vi "Demo - Advanced Use.vi"() -> ()   [LabVIEW 2013, in "GOLPI library.lvlib"]
doc: "Very simple demonstration of use of the GOLPI library.\n\n---\nGOLPI works only with lv_proc.dll library, which is part of vipm package or should be delivered together with packed library. Placement of this dll is selected in terminal of Start GNU Octave.vi."
uses:
  GOLPI library.lvlib
  Private/Set Variable - polymorph parts/Set Double Complex.vi
  Private/Get Variable - polymorph parts/Get Double.vi
panel:
  in  "octave exe file or directory":path=path "C:/Octave/Octave-4.0.0/bin"
  out "exit code of GNU\nOctave process:":i32
  out "One can see all writings to stdin or readings\nfrom stdout if debug mode was enabled:":string
  in  "timeout of this reading is":u32=14000 format="%_2p"
  out "LabVIEW now waited":u32
  in  "And wait till one of following\nkeywords appears:":string[](array[string])=["error", "demokeyword"]
  in  "Try again this time consuming\ncalculation without output:":string="for i=[1:10]\n   pause(1)\nendfor\ndisp('demokeyword')"
  out "parse error":errorcluster
  out "syntax error":errorcluster
  in  "Lets try this parse error:":string="disp()"
  in  "Lets try this syntax error:":string="sin('aa'))"
  in  "and the value of variable":string="R"
  out "LabVIEW waited":u32
  in  "timeout of all reading is":u32=14000 format="%_2p"
  in  "And read output till is settled for":u32=1200 format="%_2p"
  in  "Try this time consuming calculation:":string="for i=[1:10]\n   pause(1)\n   disp(i)\nendfor"
  out "is":dbl format="%.2f"
  in  "then calculate this equation:":string="R=abs(sqrt(Z))"
  in  "Set this value":cdb=32.56-126.3i
  in  "to a variable named":string="Z"
  out "error out":errorcluster
  in  "working directory":path=path "C:/"
  # "Writing and reading value with GOLPI Set/Get vis"
  # "How GOLPI reacts to GNU Octave syntax error"
  # ","
  # ","
  # "."
  # "Wait for GNU Octave with 'Read Output till settle.vi'"
  # "ms,"
  # "ms."
  # "ms."
  # "How GOLPI reacts to GNU Octave parse error"
  # "Wait with 'Read Output till Keyword.vi'"
  # "ms."
  # "ms."
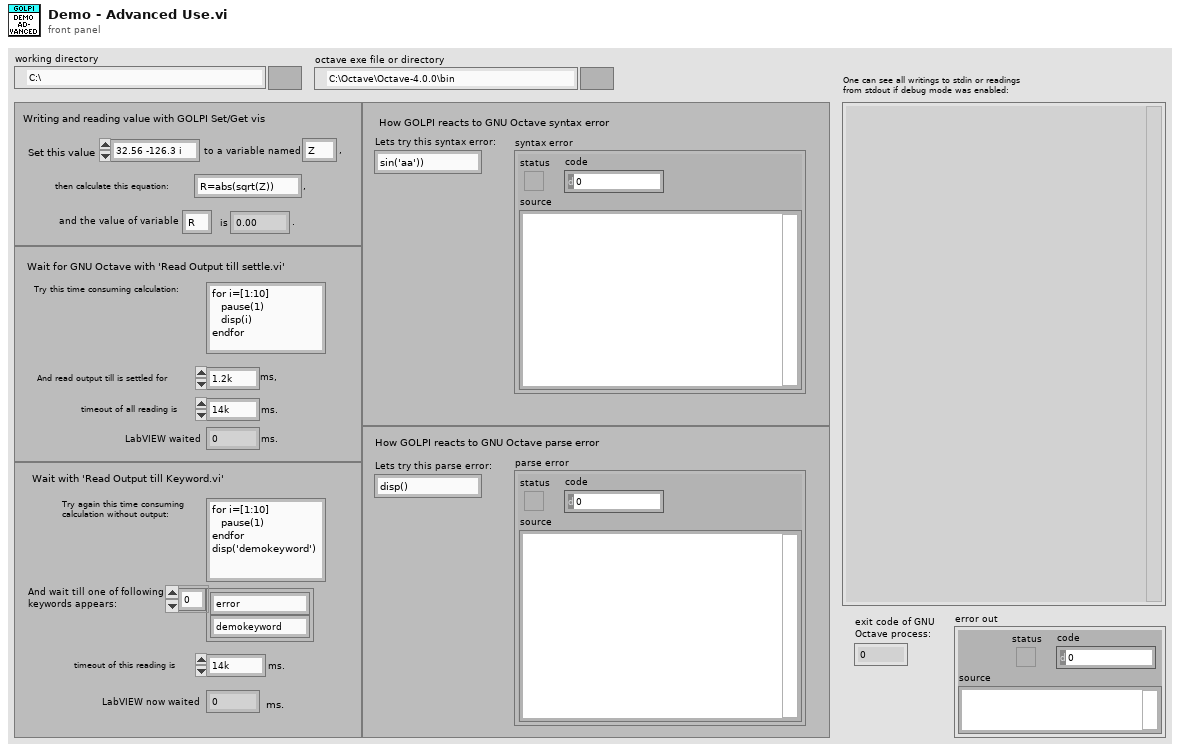
[diagram p1: front panel]
types:
  T1 = typedef "GOLPI library.lvlib/GOLPI reference Type Def.ctl" = cluster{"pipe handle":T2, "fast read timeout [ms]":u32, "fast read settle time [ms]":u32, "fast read to multiple [ms]":u32, "max elements per input line":u32, "slow read timeout [ms]":u32, "stdin double format specifier":string, "max elements per stdout output column":u32}
  T2 = typedef "LV Process library.lvlib/Pipe Handle.ctl" = cluster{"lv_proc.dll file path":path, "process instance handle":u32[], "debug mode":bool, "debug data":cluster{"time":timestamp, "stdin":bool, "data":string}[]}
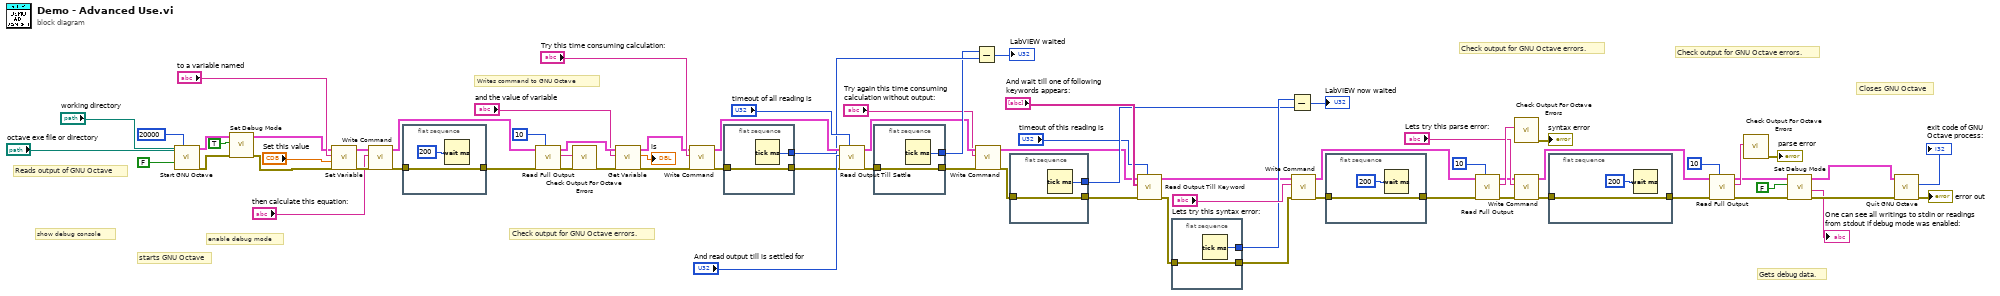
[diagram p0: block diagram]
diagram:
  # "Gets debug data."
  # "Check output for GNU Octave errors."
  # "Check output for GNU Octave errors."
  # "show debug console"
  # "enable debug mode"
  # "Check output for GNU Octave errors."
  # "Closes GNU Octave"
  # "Reads output of GNU Octave"
  # "Writes command to GNU Octave"
  # "starts GNU Octave"
  n1 = call "Start GNU Octave.vi"("working directory"="working directory", "full start timeout [ms] (20000)"=u32 20000 ("Full start timeout [ms] (5000)"), "octave exe file or directory"="octave exe file or directory", "hide debug console (T)"=FALSE) -> ("GOLPI ref. out"=w35:T1, "error out"=w3:errorcluster)  [unwired: 8 in, 2 out]
  n2 = call "Set Debug Mode.vi"("error in"=w3, "debug mode (F)"=TRUE, "GOLPI ref. in"=w35) -> ("error out"=w2:errorcluster, "GOLPI ref. out"=w34:T1)  [unwired: 5 in, 2 out]
  n3 = call-poly "Set Variable.vi"("error in"=w2, "value"="Set this value", "variable name"="to a variable named", "GOLPI ref. in"=w34) -> ("error out"=w70:errorcluster, "GOLPI ref. out"=w71:T1)  [unwired: 6 in]
  n4 = call "Write Command.vi"("error in"=w70, "command"="then calculate this equation:", "GOLPI ref. in"=w71) -> ("error out"=w28:errorcluster, "GOLPI ref. out"=w27:T1)  [unwired: 7 in]
  n5 = flat-sequence {
    tunnel: [w75] -> w29
    tunnel: w28 -> [w75]
    frame #0 {
      n6 = Wait (ms)(milliseconds to wait=u32 200) -> ()  [unwired: 1 out]
    }
  }
  n7 = call "Read Full Output.vi"("timeout [ms]"=u32 10, "error in"=w29, "GOLPI ref. in"=w27) -> ("error out"=w64:errorcluster, "read buffer"=w62:string, "GOLPI ref. out"=w63:T1)  [unwired: 5 in, 1 out]
  n8 = call "Check Output For Octave Errors.vi"("error in"=w64, "read buffer"=w62) -> ("error out"=w65:errorcluster)  [unwired: 9 in]
  n9 = call-poly "Get Variable.vi"("error in"=w65, "variable name"="and the value of variable", "GOLPI ref. in"=w63) -> ("error out"=w59:errorcluster, "value"=→"is":dbl, "GOLPI ref. out"=w58:T1)  [unwired: 6 in]
  n10 = call "Write Command.vi"("error in"=w59, "command"="Try this time consuming calculation:", "GOLPI ref. in"=w58) -> ("error out"=w54:errorcluster, "GOLPI ref. out"=w57:T1)  [unwired: 7 in]
  n11 = flat-sequence {
    tunnel: [w78] -> w53
    tunnel: w54 -> [w78]
    tunnel: [w77] -> w51
    frame #0 {
      n12 = Tick Count (ms)() -> (millisecond timer value=w77:u32)
    }
  }
  n13 = call "Read Output Till Settle.vi"("timeout [ms]"="timeout of all reading is", "error in"=w53, "settled for [ms]"="And read output till is settled for", "GOLPI ref. in"=w57) -> ("error out"=w52:errorcluster, "GOLPI ref. out"=w21:T1)  [unwired: 4 in, 2 out]
  n14 = flat-sequence {
    tunnel: [w80] -> w22
    tunnel: w52 -> [w80]
    tunnel: [w79] -> w50
    frame #0 {
      n15 = Tick Count (ms)() -> (millisecond timer value=w79:u32)
    }
  }
  n16 = Subtract(x=w50, y=w51) -> (x-y=→"LabVIEW waited":u32)
  n17 = call "Write Command.vi"("error in"=w22, "command"="Try again this time consuming\ncalculation without output:", "GOLPI ref. in"=w21) -> ("error out"=w18:errorcluster, "GOLPI ref. out"=w10:T1)  [unwired: 7 in]
  n18 = flat-sequence {
    tunnel: [w82] -> w17
    tunnel: w18 -> [w82]
    tunnel: [w81] -> w12
    frame #0 {
      n19 = Tick Count (ms)() -> (millisecond timer value=w81:u32)
    }
  }
  n20 = call "Read Output Till Keyword.vi"("timeout [ms]"="timeout of this reading is", "error in"=w17, "keywords"="And wait till one of following\nkeywords appears:", "GOLPI ref. in"=w10) -> ("error out"=w16:errorcluster, "GOLPI ref. out"=w9:T1)  [unwired: 4 in, 2 out]
  n21 = flat-sequence {
    tunnel: [w84] -> w15
    tunnel: w16 -> [w84]
    tunnel: [w83] -> w13
    frame #0 {
      n22 = Tick Count (ms)() -> (millisecond timer value=w83:u32)
    }
  }
  n23 = Subtract(x=w13, y=w12) -> (x-y=→"LabVIEW now waited":u32)
  n24 = call "Write Command.vi"("error in"=w15, "command"="Lets try this syntax error:", "GOLPI ref. in"=w9) -> ("error out"=w26:errorcluster, "GOLPI ref. out"=w44:T1)  [unwired: 7 in]
  n25 = flat-sequence {
    tunnel: [w85] -> w25
    tunnel: w26 -> [w85]
    frame #0 {
      n26 = Wait (ms)(milliseconds to wait=u32 200) -> ()  [unwired: 1 out]
    }
  }
  n27 = call "Read Full Output.vi"("timeout [ms]"=u32 10, "error in"=w25, "GOLPI ref. in"=w44) -> ("error out"=w40:errorcluster, "read buffer"=w45:string, "GOLPI ref. out"=w8:T1)  [unwired: 5 in, 1 out]
  n28 = call "Check Output For Octave Errors.vi"("read buffer"=w45) -> ("error out"=→"syntax error":errorcluster)  [unwired: 10 in]
  n29 = call "Write Command.vi"("error in"=w40, "command"="Lets try this parse error:", "GOLPI ref. in"=w8) -> ("error out"=w24:errorcluster, "GOLPI ref. out"=w43:T1)  [unwired: 7 in]
  n30 = flat-sequence {
    tunnel: [w87] -> w23
    tunnel: w24 -> [w87]
    frame #0 {
      n31 = Wait (ms)(milliseconds to wait=u32 200) -> ()  [unwired: 1 out]
    }
  }
  n32 = call "Read Full Output.vi"("timeout [ms]"=u32 10, "error in"=w23, "GOLPI ref. in"=w43) -> ("error out"=w7:errorcluster, "read buffer"=w42:string, "GOLPI ref. out"=w32:T1)  [unwired: 5 in, 1 out]
  n33 = call "Check Output For Octave Errors.vi"("read buffer"=w42) -> ("error out"=→"parse error":errorcluster)  [unwired: 10 in]
  n34 = call "Set Debug Mode.vi"("error in"=w7, "debug mode (F)"=FALSE, "GOLPI ref. in"=w32) -> ("error out"=w6:errorcluster, "debug data strings concatenated"=→"One can see all writings to stdin or readings\nfrom stdout if debug mode was enabled:":string, "GOLPI ref. out"=w31:T1)  [unwired: 5 in, 1 out]
  n35 = call "Quit GNU Octave.vi"("error in"=w6, "GOLPI ref. in"=w31) -> ("error out"=→"error out":errorcluster, "exit code"=→"exit code of GNU\nOctave process:":i32)  [unwired: 8 in]
